vi "Save As Tiff Ex.vi"(6 "mode":i32, 7 "typ":i32, 8 "error in (no error)":errorcluster, 9 "position":i32, 10 "palette":string, 11 "path":string) -> (0 "error out":errorcluster, 1 "function return":u32, 2 "palette out":string, 3 "path out":string)   [LabVIEW 2014, in "atmcd32d.lvlib"]
doc: "unsigned int WINAPI SaveAsTiffEx(char * path, char * palette, int position, int typ, int mode);"
uses:
  atmcd32d.lvlib
  atmcd32d.dll
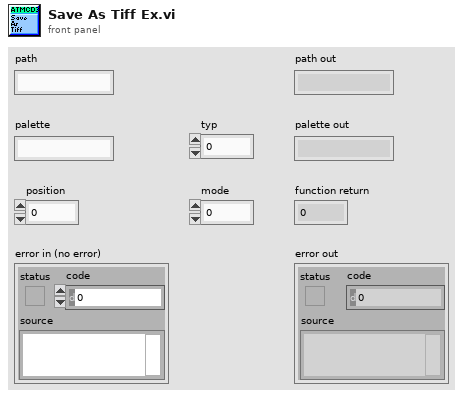
[diagram p1: front panel]
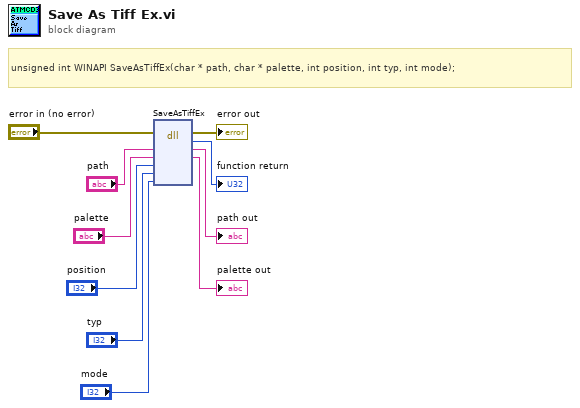
[diagram p0: block diagram]
diagram:
  # "unsigned int WINAPI SaveAsTiffEx(char * path, char * palette, int position, int typ, int mode);"
  n1 = dll-call lib="C:/Users/Bakir/Documents/Lambda2-Testing/lib/Andorlib/atmcd32d.*" fn="SaveAsTiffEx"(error in="error in (no error)", "path"="path", "palette"="palette", "position"="position", "typ"="typ", "mode"="mode") -> (error out=→"error out":errorcluster, →"function return":u32, "path"=→"path out":string, "palette"=→"palette out":string)  [unwired: 5 in, 1 out]
